vi "create_file_sin (SubVI).vi"(0 "Channel":i32, 1 "Trigger Width":dbl format="%#_13g", 4 "Frequency (MHz)":dbl, 5 "Square Pulse Amplitude":dbl format="%#_13g", 6 "Amplitude":dbl, 7 "Pulse Width":dbl, 8 "Number Of Points(integer multiple of 4096)":i32, 9 "DAC frequency (MHz)":dbl, 10 "Pulse Center":dbl format="%#_13g", 11 "file path (use dialog)":path) -> (2 "output waveform 2":waveform(dbl)(graph), 3 "output waveform":waveform(dbl)(graph))   [LabVIEW 2016]
panel:
  out "x <= y?":bool
  out "x-y":dbl
  out "Array":i32[](array[numeric])
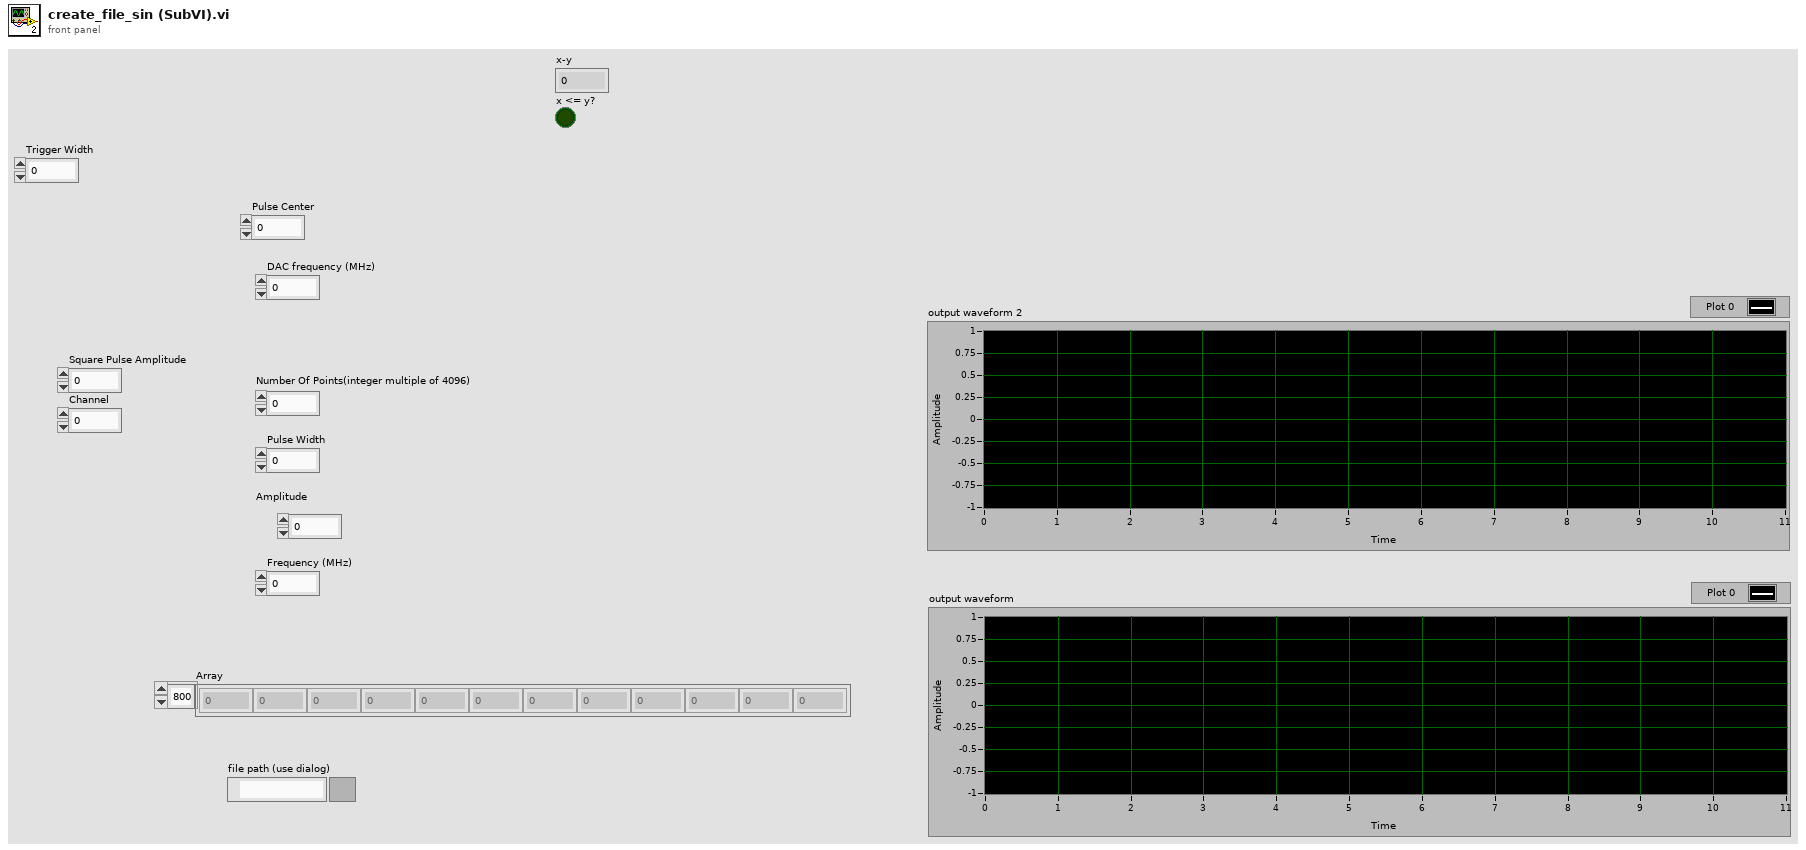
[diagram p1: front panel]
types:
  T1 = enum16{"open", "replace", "create", "open or create", "replace or create", "replace or create with confirmation"}
  T2 = enum16{"big-endian, network order", "native, host order", "little-endian"}
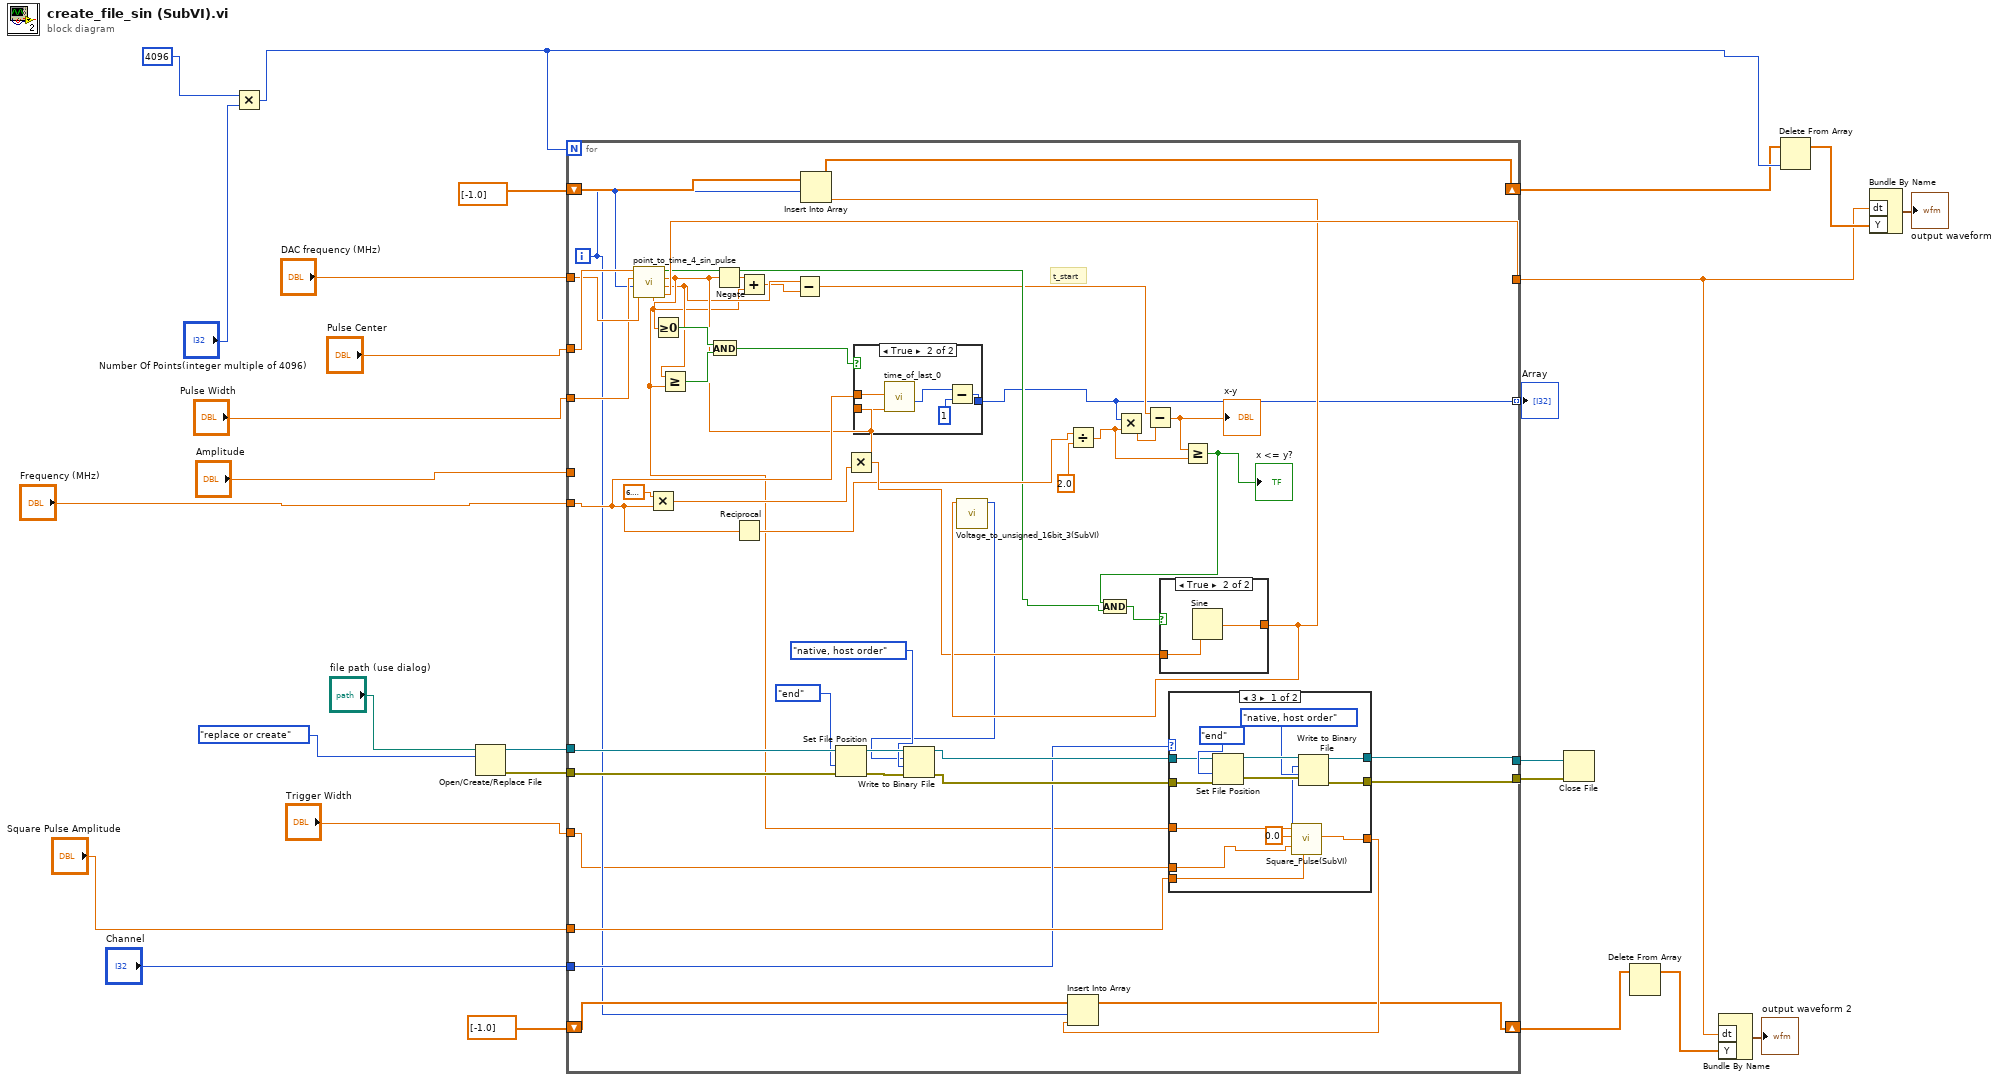
[diagram p0: block diagram]
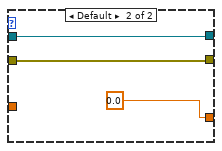
[diagram p2: hidden frame]
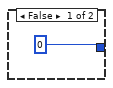
[diagram p3: hidden frame]
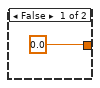
[diagram p4: hidden frame]
diagram:
  n1 = Multiply(x=4096, y="Number Of Points(integer multiple of 4096)") -> (x*y=w27:i32)
  n2 = Open/Create/Replace File(file path (use dialog)="file path (use dialog)", operation (0:open)=T1."replace or create") -> (refnum out=w14:refnum<file>, error out=w13:errorcluster)  [unwired: 4 in, 1 out]
  n3 = for {
    N: w27 -> [_]
    tunnel: "Amplitude" -> [_]
    shift-right: [w73] -> w26
    shift-left: dbl[] [-1.0] ("array") -> [w74]
    tunnel: "Frequency (MHz)" -> [w60]
    tunnel: "DAC frequency (MHz)" -> [w69]
    tunnel: [w71] -> w4
    tunnel: "Pulse Center" -> [w70]
    tunnel: "Pulse Width" -> [w68]
    tunnel: [w47] -> w17 mode=indexing
    tunnel: w14 -> [w44]
    tunnel: w13 -> [w42]
    tunnel: [w37] -> w12
    tunnel: [w36] -> w11
    tunnel: "Square Pulse Amplitude" -> [w35]
    tunnel: "Channel" -> [w34]
    shift-right: [w30] -> w2
    shift-left: dbl[] [-1.0] ("array") -> [w33]
    tunnel: "Trigger Width" -> [w28]
    i -> [w32]
    # "t_start"
    n4 = call "point_to_time_4_sin_pulse.vi"("DAC frequency(MHz)"=w69, "point location"=w32, "Pulse Width"=w68, "Pulse Center (us)"=w70) -> ("dt (us)"=w71:dbl, "t_finish"=w50:dbl, "t - t_start"=w52:dbl, "t inside pulse width"=w54:bool, "t"=w29:dbl)  [unwired: 3 in]
    n5 = Multiply(x=6.283185307179586, y=w60) -> (x*y=w62:dbl)
    n6 = Greater Or Equal To 0?(x=w52) -> (x >= 0?=w65:bool)
    n7 = Greater Or Equal?(x=w50, y=w29) -> (x >= y?=w64:bool)
    n8 = And(x=w65, y=w64) -> (x .and. y?=w63:bool)
    n9 = Negate(x=w52) -> (-x=w51:dbl)
    n10 = Reciprocal(x=w60) -> (1/x=w58:dbl)
    n11 = Add(x=w51, y=w29) -> (x+y=w49:dbl)
    n12 = Subtract(x=w50, y=w49) -> (x-y=w48:dbl)
    n13 = Set File Position(refnum=w44, from (0:start)=enum16{"start", "end", "current"}."end", error in=w42) -> (refnum out=w45:refnum<file>, error out=w46:errorcluster)  [unwired: 1 in]
    n14 = Multiply(x=w52, y=w62) -> (x*y=w66:dbl)
    n15 = case shown="True" w63 {
      tunnel: w60 -> [_ w97]
      tunnel: w52 -> [_ w96]
      tunnel: [0 w93] -> w47
      frame False {
      }
      frame True {
        n16 = call "time_of_last_0.vi"("time"=w96, "Frequency (Hz)"=w97) -> ("Number of zeroes"=w95:i32)  [unwired: 8 in, 1 out]
        n17 = Subtract(x=w95, y=1) -> (x-y=w93:i32)
      }
    }
    n18 = Divide(x=w58, y=2.0) -> (x/y=w56:dbl)
    n19 = Multiply(x=w47, y=w56) -> (x*y=w61:dbl)
    n20 = Subtract(x=w48, y=w61) -> (x-y=w57:dbl)
    "x-y" <- w57
    n21 = Greater Or Equal?(x=w57, y=w56) -> (x >= y?=w55:bool)
    "x <= y?" <- w55
    n22 = And(x=w55, y=w54) -> (x .and. y?=w53:bool)
    n23 = case shown="True" w53 {
      tunnel: w66 -> [_ w100]
      tunnel: [0.0 w99] -> w67
      frame False {
      }
      frame True {
        n24 = Sine(x=w100) -> (sin(x)=w99:dbl)
      }
    }
    n25 = Insert Into Array(array=w74, index=w32, new element=w67) -> (w73:dbl[])
    n26 = call "Voltage_to_unsigned_16bit_3(SubVI).vi"("Voltage_in"=w67) -> ("unsigned 16bit integer"=w40:u16)  [unwired: 10 in]
    n27 = Write to Binary File(file (use dialog)=w45, data=w40, error in=w46, 9:T2."native, host order" ("byte order (0:big-endian, network order)")) -> (refnum out=w39:refnum<file>, error out=w38:errorcluster)  [unwired: 2 in, 1 out]
    n28 = case shown="3" w34 {
      tunnel: w35 -> [w88 _]
      tunnel: [w87 0.0] -> w31
      tunnel: w28 -> [w75 _]
      tunnel: w38 -> [w85 w91]
      tunnel: [w82 w90] -> w37
      tunnel: [w81 w91] -> w36
      tunnel: w39 -> [w78 w90]
      tunnel: w29 -> [w77 _]
      frame 3 {
        n29 = Set File Position(refnum=w78, from (0:start)=enum16{"start", "end", "current"}."end", error in=w85) -> (refnum out=w84:refnum<file>, error out=w83:errorcluster)  [unwired: 1 in]
        n30 = call "Square_Pulse(SubVI).vi"("High Voltage (V)"=w88, "Pulse Width"=w75, "Pulse Start (us)"=0.0, "Time"=w77) -> ("Voltage Out"=w87:dbl, "unsigned 16-bit out"=w79:u16)  [unwired: 6 in]
        n31 = Write to Binary File(file (use dialog)=w84, data=w79, error in=w83, 9:T2."native, host order" ("byte order (0:big-endian, network order)")) -> (refnum out=w82:refnum<file>, error out=w81:errorcluster)  [unwired: 2 in, 1 out]
      }
      frame Default {
      }
    }
    n32 = Insert Into Array(array=w33, index=w32, new element=w31) -> (w30:dbl[])
  }
  "Array" <- w17
  n33 = Close File(refnum=w12, error in=w11) -> ()  [unwired: 2 out]
  n34 = Delete From Array(array=w2) -> (array with subset deleted=w6:dbl[])  [unwired: 2 in, 1 out]
  n35 = Bundle By Name("dt"=w4, "Y"=w6) -> (→"output waveform 2":waveform(dbl))  [unwired: 1 in]
  n36 = Delete From Array(array=w26, index=w27) -> (array with subset deleted=w25:dbl[])  [unwired: 1 in, 1 out]
  n37 = Bundle By Name("dt"=w4, "Y"=w25) -> (→"output waveform":waveform(dbl))  [unwired: 1 in]
